vi "franch_freq_offset_correction.vi"(9 "freq offset":dbl, 11 "input signal":cdb[](array[numeric])) -> (3 "Corrected Signal":cdb[](array[numeric]))   [LabVIEW 2012]
uses:
  <vilib>/Analysis/1siggen.llb/Ramp Pattern by Samples.vi
  <vilib>/Analysis/NI_AALBase.lvlib
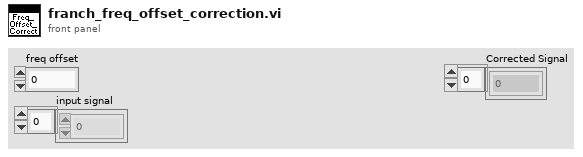
[diagram p1: front panel]
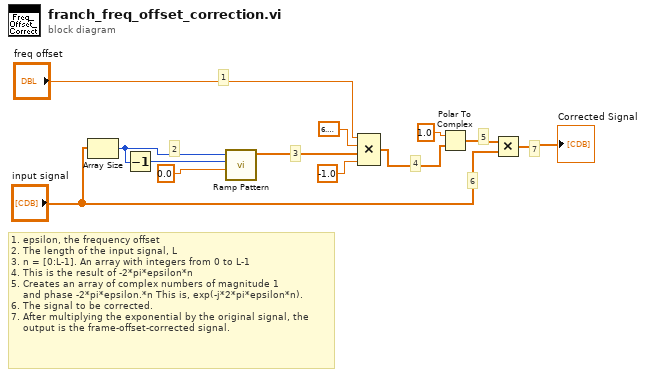
[diagram p0: block diagram]
diagram:
  # "1. epsilon, the frequency offset\n2. The length of the input signal, L\n3. n = [0:L-1]. An array with integers from 0 to L-1\n4. This is the result of -2*pi*epsilon*n\n5. Creates an array of complex numbers of magnitude 1\n    and phase -2*pi*epsilon.*n This is, exp(-j*2*pi*epsilon*n).\n6. The signal to be corrected.\n7. After multiplying the exponential by the original signal, the\n    output is the frame-offset-corrected signal."
  # "7"
  # "6"
  # "5"
  # "4"
  # "3"
  # "2"
  # "1"
  n1 = Array Size(array="input signal") -> (size(s)=w10:i32)
  n2 = Decrement(x=w10) -> (x-1=w12:i32)
  n3 = call-poly <vilib>:"Ramp Pattern.vi"("start"=0.0, "end"=w12, "samples"=w10) -> ("Ramp Pattern"=w7:dbl[])  [unwired: 7 in, 1 out]
  n4 = Compound Arithmetic op=MULTIPLY("freq offset", 6.283185307179586, w7, -1.0 ("start")) -> (w1:dbl[])
  n5 = Polar To Complex(1:w1, 2:1.0 ("element")) -> (0:w9:cdb[])
  n6 = Multiply(x=w9, y="input signal") -> (x*y=→"Corrected Signal":cdb[])
